vi "torsional-interface-template.vi"() -> ()   [LabVIEW 2013]
doc: "This is a template VI for interfacing with the ECP Torsional Plant using an FPGA card."
uses:
  <vilib>/Simulation/Scripting/Companion Diagram/SimConfigNode/SimParams.ctl
  <vilib>/Simulation/Scripting/Companion Diagram/SimConfigNode/_simSolvers.ctl
  <vilib>/Simulation/Implementation/Shared/SIMSCR Execution Mode.ctl
  <vilib>/Platform/TimedLoop/XDataNode/timing_clust.ctl
  <vilib>/Platform/TimedLoop/XDataNode/nitl_modes.ctl
  <vilib>/Platform/TimedLoop/XDataNode/wakeup.ctl
  <vilib>/Simulation/Param Hierarchy/Typedefs/SIMPH Param Control Actions.ctl
  <vilib>/Simulation/Scripting/Editor Utilities/SIM subVI tag data.ctl
  <vilib>/Simulation/Scripting/Editor Utilities/SIM subVI execution type.ctl
  <vilib>/Simulation/Implementation/Shared/NILVSim_ParamChanged.vi
  <vilib>/Simulation/Implementation/Shared/NILVSim_FinishedLate.vi
  <vilib>/Simulation/Implementation/Shared/NILVSIM_BeginStep.vi
  <vilib>/Simulation/Utility/Implementation/SIM Halt.vi
  <vilib>/Simulation/Implementation/Shared/SIM Fire Discrete SubVI.vi
  <vilib>/Simulation/SignalArithmetic/Implementation/NILVSim Gain.llb/SIM Gain (scalar).vi
  <vilib>/Simulation/SignalDisplay/Implementation/NILVSim Time Waveform.llb/SIM Time Waveform (scalar).vi
  <vilib>/Simulation/SignalArithmetic/Implementation/NILVSim Gain.llb/SIM Gain (vector).vi
  <vilib>/Simulation/SignalDisplay/Implementation/NILVSim Time Waveform.llb/SIM Time Waveform (vector).vi
  <vilib>/Simulation/Implementation/Shared/NILVSim_Manager.vi
  <vilib>/Simulation/Implementation/Shared/NILVSim_FinalizeModel.vi
  <vilib>/Simulation/Implementation/Shared/SIM Fire Discrete SubVI (Core).vi
  <vilib>/FPGAPlugInAG/PCI-7831R/niLvFpga_Open_PCI-7831R.vi
  <vilib>/FPGAPlugInAG/PCI-7831R/niLvFpga_Download_PCI-7831R.vi
  <vilib>/FPGAPlugInAG/PCI-7831R/niLvFpga_Run_PCI-7831R.vi
  <vilib>/Utility/error.llb/Error Cluster From Error Code.vi
  <vilib>/rvi/errors/niLvFpgaAdjustHostInterfaceError.vi
  <vilib>/Simulation/Implementation/Shared/SIM Unbundle Sim Info.vi
  <vilib>/Utility/error.llb/Clear Errors.vi
  <vilib>/Simulation/Implementation/Shared/NILVSim_GetModelError.vi
  <vilib>/Simulation/Implementation/Shared/SIM Bundle Sim Info.vi
  <vilib>/Simulation/Implementation/Shared/SIMSH Read Queue.vi
  <vilib>/Simulation/Implementation/Shared/NILVSim_Initialize.vi
  <vilib>/Simulation/Utility/Implementation/NILVSim Get Time and IsAcceptedStep.vi
  <vilib>/FPGAPlugInAG/PCI-7831R/niLvFpga_Close_PCI-7831R.vi
  <vilib>/rvi/interface/nirviOpenFPGA/nirviOpenFPGA.xnode
  torsional-fpga-interface.lvbitx
  <vilib>/rvi/interface/nirviMethod/nirviMethod.xnode
  <vilib>/rvi/interface/nirviReadWriteControl/nirviReadWriteControl.xnode
  <vilib>/Simulation/Scripting/Companion Diagram/SimConfigNode/SimDog.xnode
  <vilib>/Simulation/Model Libraries/PID/SIM PID (Parallel).vi
  <vilib>/Simulation/Model Libraries/PID/SIM PID.vi
  <vilib>/Platform/TimedLoop/XDataNode/XDataNode.xnode
  <vilib>/Simulation/Implementation/XNodeFramework/SimXNode/SimX.xnode
  <vilib>/rvi/interface/nirviCloseFPGA/nirviCloseFPGA.xnode
  NiFpgaLv.dll
  <vilib>/Platform/TimedLoop/XDataNode/XDNodeRunTimeDep.lvlib
  <vilib>/Simulation/Implementation/Shared/NI_SIM_Implementation.lvlib
panel:
  out "output":dbl[](array[numeric])
  out "Waveform Chart 2":waveform(dbl)(graph)
  out "Waveform Chart":waveform(dbl)[](graph)
  out "Killswitch\nActivated":bool
  out "Sample Rate (Hz)":dbl
  in  "Abort":bool
  in  "Final Time (s)":dbl=30.0 min=0.0 step=0.01
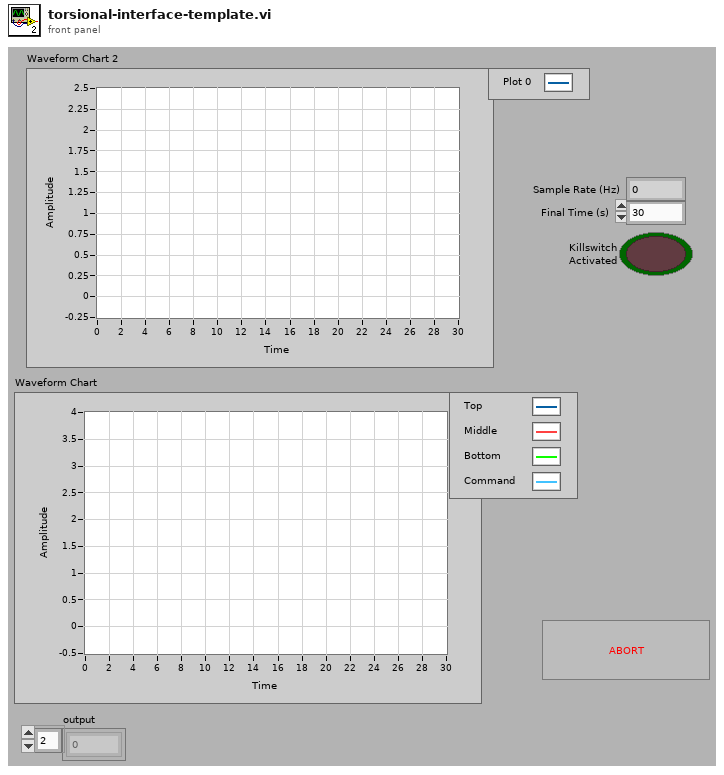
[diagram p1: front panel]
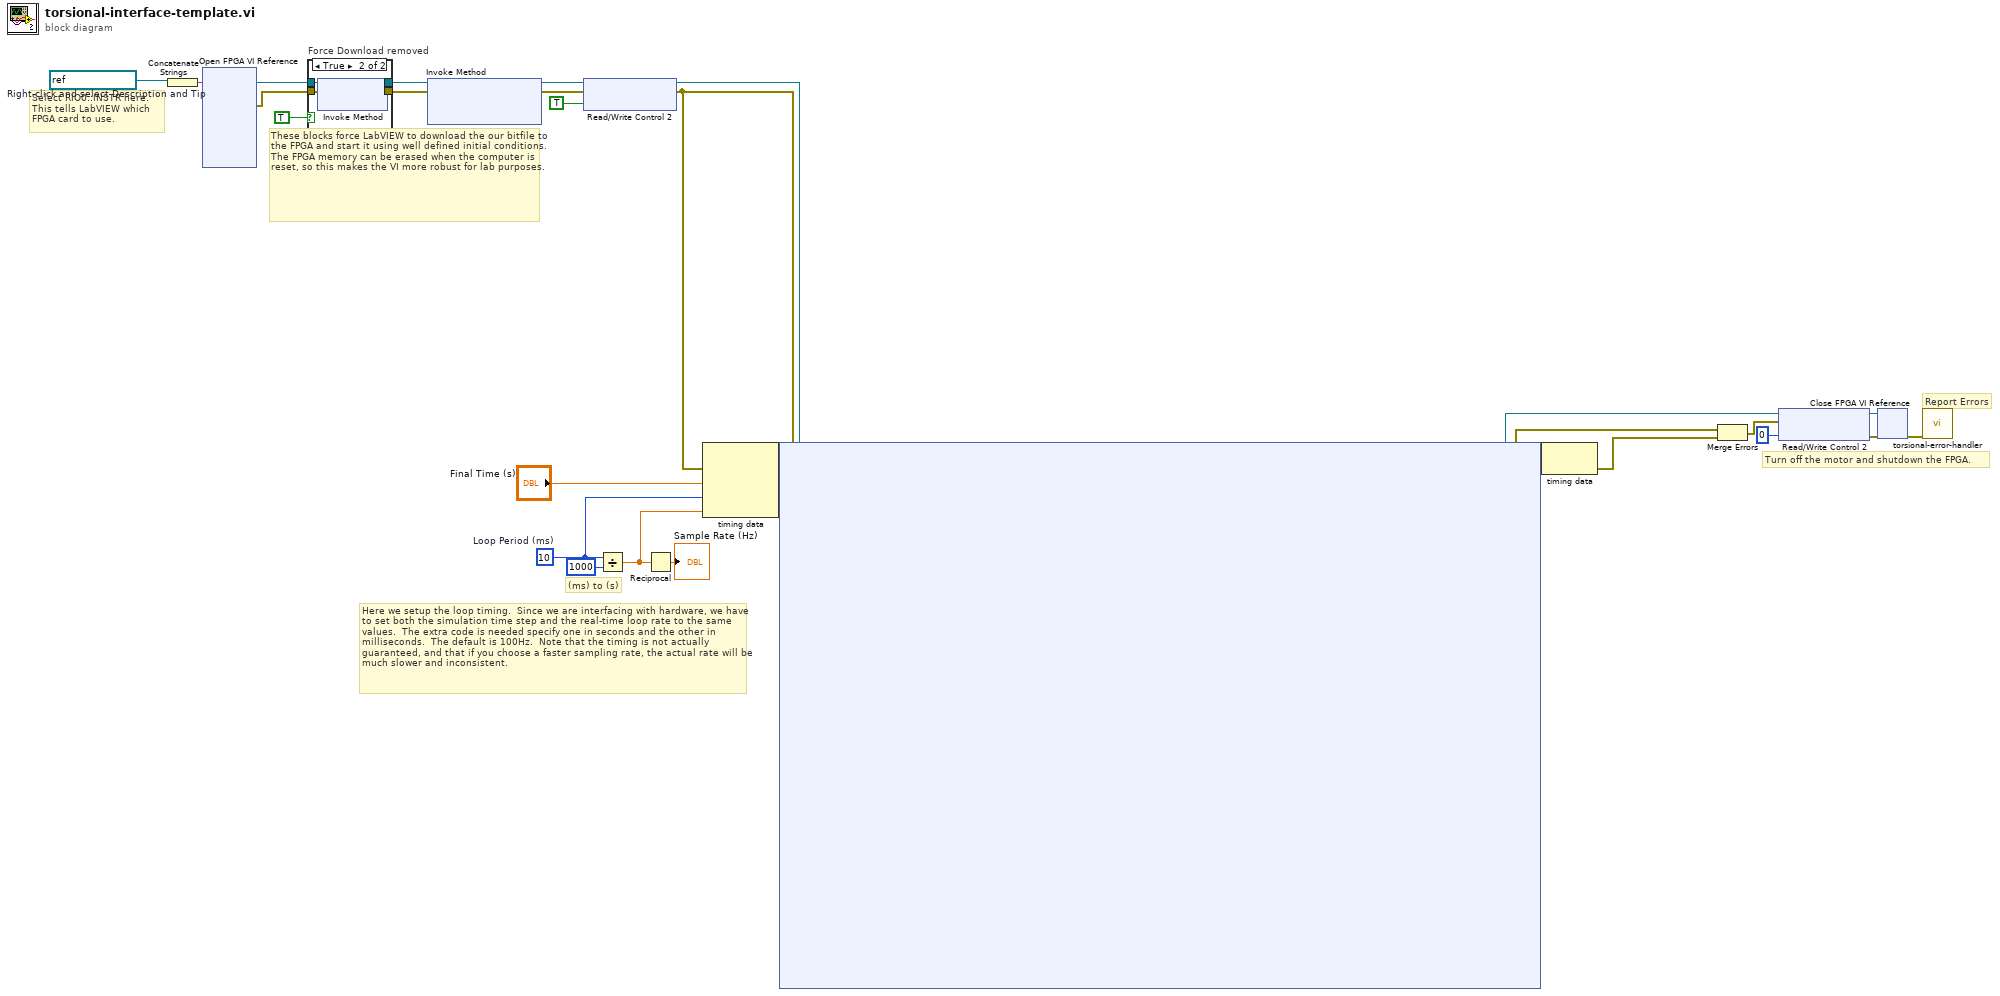
[diagram p0: block diagram]
diagram:
  w3 = 10  # Loop Period (ms)
  # "(ms) to (s)"
  # "Report Errors"
  # "Here we setup the loop timing.  Since we are interfacing with hardware, we have to set both the simulation time step and the real-time loop rate to the same values.  The extra code is needed specify one in seconds and the other in milliseconds.  The default is 100Hz.  Note that the timing is not actually guaranteed, and that if you choose a faster sampling rate, the actual rate will be much slower and inconsistent."
  # "These blocks force LabVIEW to download the our bitfile to the FPGA and start it using well defined initial conditions.  The FPGA memory can be erased when the computer is reset, so this makes the VI more robust for lab purposes."
  # "Turn off the motor and shutdown the FPGA."
  # "Select RIO0::INSTR here.  This tells LabVIEW which FPGA card to use."
  n1 = Concatenate Strings "Right-click and select Description and Tip"(refnum<visa-resource-name> "RIO0::INSTR" ("resource name")) -> (w1:string)
  n2 = xnode "Open FPGA VI Reference"("resource name"=w1) -> ("FPGA VI Reference Out"=w16:refnum<k20>, "error out"=w22:errorcluster)  [unwired: 1 in]
  n3 = case "Force Download removed" shown="True" TRUE ("Force Download (F)") {
    tunnel: w16 -> [w29 w33]
    tunnel: [w29 w32] -> w15
    tunnel: w22 -> [w28 w31]
    tunnel: [w28 w30] -> w13
    frame False {
    }
    frame True {
      n4 = xnode "Invoke Method"("FPGA VI Reference In"=w33, "error in"=w31) -> ("FPGA VI Reference Out"=w32:refnum<k20>, "error out"=w30:errorcluster)
    }
  }
  n5 = xnode "Invoke Method"("FPGA VI Reference In"=w15, "error in"=w13) -> ("FPGA VI Reference Out"=w25:refnum<k20>, "error out"=w21:errorcluster)  [unwired: 1 in]
  n6 = xnode ("Read/Write Control 2")("FPGA VI Reference In"=w25, "error in"=w21, "Reset Encoders"=TRUE) -> ("FPGA VI Reference Out"=w11:refnum<k20>, "error out"=w6:errorcluster)
  n7 = Divide(x=w3, y=1000) -> (x/y=w2:dbl)
  n8 = Reciprocal(x=w2) -> (1/x=→"Sample Rate (Hz)":dbl)
  n9 = node-c288(w6, "Final Time (s)", w3, w2) -> (w27:variant)
  n10 = node-c254 ("Control & Simulation Loop")(w27, w6, w11) -> (w26:variant, w9:refnum<k20>, w8:errorcluster)
  n11 = node-c288(w26) -> (w7:errorcluster)
  n12 = Merge Errors(w8, w7) -> (w10:errorcluster)
  n13 = xnode ("Read/Write Control 2")("FPGA VI Reference In"=w9, "error in"=w10, "Motor Voltage"=i16 0 ("Analog Out")) -> ("FPGA VI Reference Out"=w20:refnum<k20>, "error out"=w18:errorcluster)
  n14 = xnode ("Close FPGA VI Reference")("FPGA VI Reference In"=w20, "error in"=w18) -> ("error out"=w17:errorcluster)
  n15 = call "torsional-error-handler.vi"("error in"=w17) -> ()  [unwired: 4 in]
